vi "Write_to_log_file.vi"(6 "User added comment":string, 8 "End time":dbl format="%.2f", 9 "Start time":dbl format="%.2f", 11 "Folder/file":path) -> (0 "File Updated?":bool)   [LabVIEW 2015]
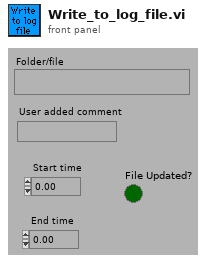
[diagram p1: front panel]
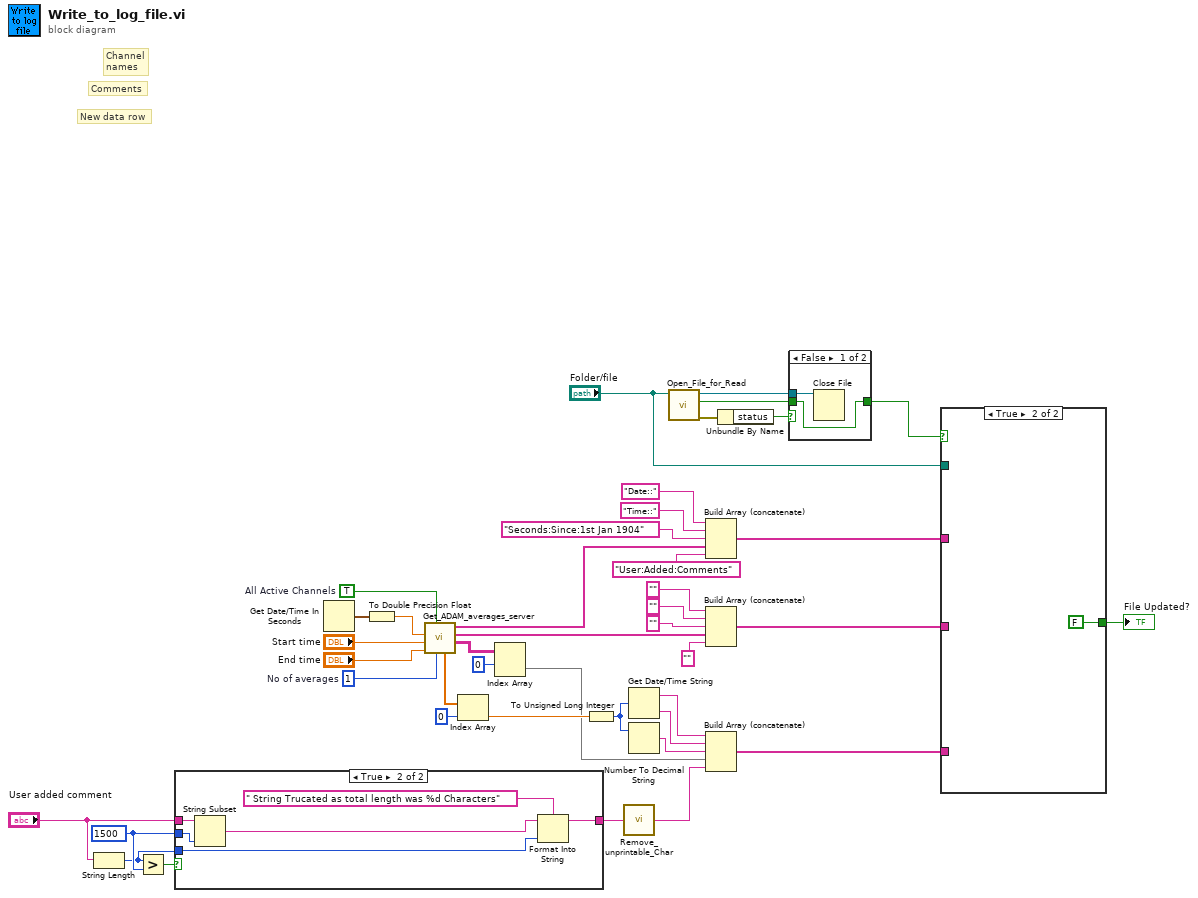
[diagram p0: block diagram]
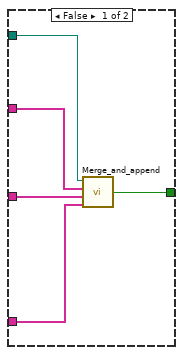
[diagram p2: hidden frame]
diagram:
  w22 = 1500 ("y")
  w30 = 1  # No of averages
  w34 = TRUE  # All Active Channels
  # "Comments"
  # "New data row"
  # "Channel\nnames"
  n1 = String Length(string="User added comment") -> (length=w21:i32)
  n2 = Greater?(x=w21, y=w22) -> (0:w24:bool)
  n3 = case shown="True" w24 {
    tunnel: [w43 w44] -> w38
    tunnel: "User added comment" -> [w43 w49]
    tunnel: w22 -> [_ w45]
    tunnel: w21 -> [_ w48]
    frame False {
    }
    frame True {
      n4 = String Subset(string=w49, length (rest)=w45) -> (substring=w47:string)  [unwired: 1 out]
      n5 = Format Into String(format string=" String Trucated as total length was %d Characters", initial string=w47, w48) -> (resulting string=w44:string)  [unwired: 1 in, 1 out]
    }
  }
  n6 = Get Date/Time In Seconds() -> (seconds since 1Jan1904=w25:timestamp)
  n7 = To Double Precision Float(number=w25) -> (double precision float=w33:dbl)
  n8 = call "Get_ADAM_averages_server.vi"("No of averages"=w30, "All Active Channels"=w34, "End time"="End time", "Start time"="Start time", "Clients time"=w33) -> ("Values"=w26:string[][], "Comments"=w42:string[], "Titles"=w41:string[], "Times"=w28:dbl[])  [unwired: 1 in, 1 out]
  n9 = Index Array(array=w28, index=0 ("Index")) -> (element=w40:dbl)
  n10 = Index Array(array=w26, index (row)=0) -> (element=w39:string[])  [unwired: 1 in]
  n11 = To Unsigned Long Integer(number=w40) -> (unsigned 32bit integer=w9:u32)
  n12 = call "Remove_unprintable_Char.vi"("Input String"=w38) -> ("Output String"=w8:string)
  n13 = Get Date/Time String(seconds (now)=w9) -> (date string=w12:string, time string=w11:string)  [unwired: 2 out]
  n14 = Number To Decimal String(number=w9) -> (decimal integer string=w10:string)  [unwired: 1 out]
  n15 = call "Open_File_for_Read.vi"("file path"="Folder/file") -> ("error out"=w6:errorcluster, "Permission error?"=w2:bool, "refnum"=w4:refnum<file>)  [unwired: 8 out]
  n16 = Build Array (concatenate)("Date::", "Time::", "Seconds:Since:1st Jan 1904", w41, "User:Added:Comments") -> (w37:string[])
  n17 = Build Array (concatenate)("", "", "", w42, "") -> (w35:string[])
  n18 = Build Array (concatenate)(w12, w11, w10, w39, w8) -> (w36:string[])
  n19 = Unbundle By Name(w6) -> ("status"=w5:bool)
  n20 = case shown="False" w5 {
    tunnel: w4 -> [w51 _]
    tunnel: [w50 w52] -> w1
    tunnel: w2 -> [w50 w52]
    frame False {
      n21 = Close File(refnum=w51) -> ()  [unwired: 1 in, 2 out]
    }
    frame True {
    }
  }
  n22 = case shown="True" w1 {
    tunnel: w37 -> [w57 _]
    tunnel: w35 -> [w56 _]
    tunnel: w36 -> [w55 _]
    tunnel: [w54 FALSE ("File Updated?")] -> w7
    tunnel: "Folder/file" -> [w53 _]
    frame False {
      n23 = call "Merge_and_append.vi"("New Row"=w55, "Comments"=w56, "Channel Names"=w57, "Path name"=w53) -> ("File Updated?"=w54:bool)
    }
    frame True {
    }
  }
  "File Updated?" <- w7
